vi "Main Data Log.vi"(8 "error in (no error)":errorcluster, 11 "main ref":T1) -> (0 "error out":errorcluster)   [LabVIEW 2025]
uses:
  controls/LAB-IQ UI Data.ctl
panel:
  out "error out 2":errorcluster
  out "TDMS CLOSE":bool
  out "tdms file out":refnum<k34>
  out "File Create Temp":bool
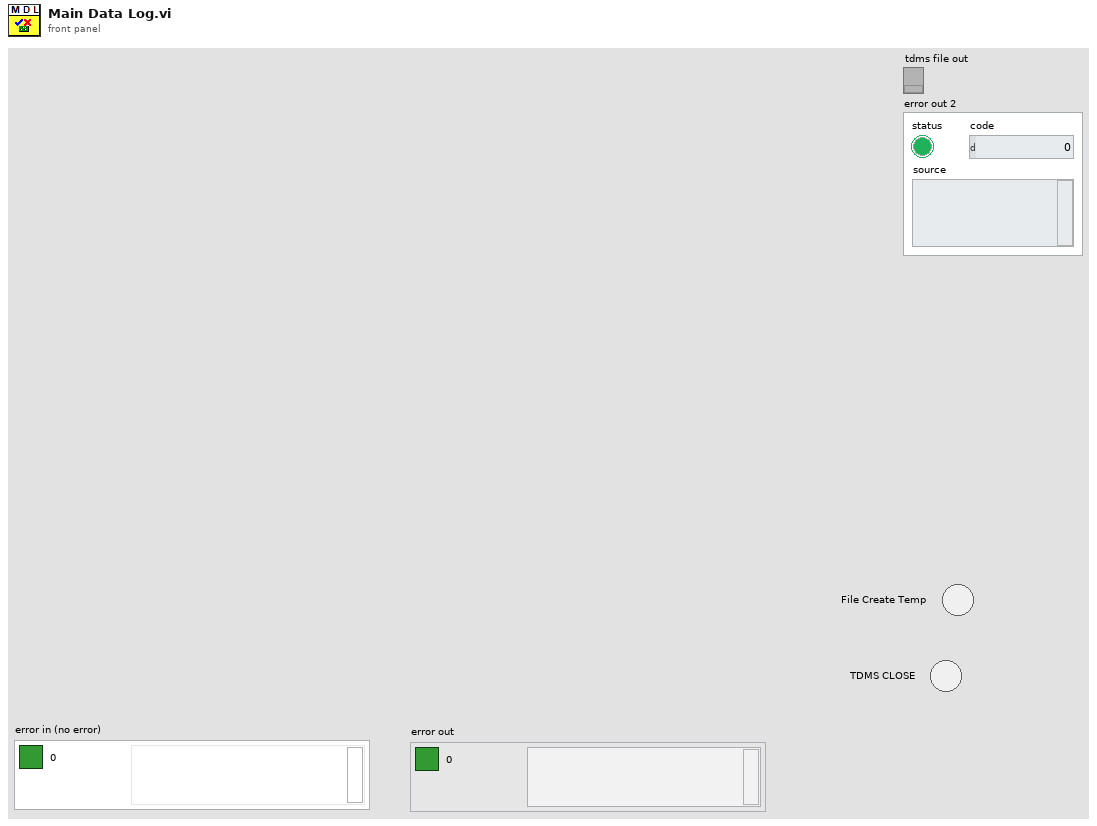
[diagram p1: front panel]
types:
  T1 = typedef "LAB-IQ UI Data.ctl" = cluster{"Main Home Screen":cluster{"GUI":refnum<vi>, "Platform Settings":refnum<vi>, "Configure":refnum<vi>, "Home":refnum<vi>, "EXIT":refnum<vi>, "service 2":refnum<vi>, "MainPage":refnum<vi>, "Analysis":refnum<vi>}, "Platform Settings":cluster{"mm/s  Surge":refnum<vi>, "Update Surge Speed":refnum<vi>, "Drive Error":refnum<vi>, "Disable Axis Jog Soft Limits":refnum<vi>, "mm/s  Sway":refnum<vi>, "Sway and Surge COM Status":refnum<vi>, "Heave COM Status":refnum<vi>, "Enable Platform":refnum<vi>, "Surge Forward Main":refnum<vi>, "Sway Right Main":refnum<vi>, "Sway Left Main":refnum<vi>, "Heave Down Main":refnum<vi>, "Heave Up main":refnum<vi>, "Update Sway Speed":refnum<vi>, "Update Heave Speed":refnum<vi>, "mm/s Heave":refnum<vi>, "mm/sec":refnum<vi>, "mm":refnum<vi>, "Surge Backward Main":refnum<vi>}, "Analysis Screen":cluster{"Analysis Home":refnum<vi>, "Surface Analysis":refnum<vi>, "Imaging":refnum<vi>, "Image Analysis":refnum<vi>, "Post Analysis":refnum<vi>}, "Config Screen":cluster{"Select Load Head":refnum<vi>, "Notes :":refnum<vi>, "FILE":refnum<vi>, "Sample ID :":refnum<vi>, "Operator ID :":refnum<vi>, "Operator Name :":refnum<vi>, "Auto":refnum<vi>}, "Motion Module":cluster{"zNL":refnum<vi>, "NL disp":refnum<vi>, "Rotary Tab":refnum<vi>, "Motion Direction:  3":refnum<vi>, "E.Velocity 2":refnum<vi>, "e.v/ssr 2":refnum<vi>, "Enter Fixed E.Velocity 2":refnum<vi>, "Enter Final SRR 2":refnum<vi>, "Enter initial SRR 2":refnum<vi>, "Enter Fixed SRR 2":refnum<vi>, "Enter the Final E.Velocity (m/s) 2":refnum<vi>, "Enter initial E.Velocity (m/s) 2":refnum<vi>, "Final Speed (RPM) 3":refnum<vi>, "Initial Speed (RPM) 2":refnum<vi>, "Enter the Final Velocity (m/s) 3":refnum<vi>, "Enter initial Velocity (m/s)  3":refnum<vi>, "Ramp Up 2":refnum<vi>, "TEST SELECTION":refnum<vi>, "SPEED SELECTION : ":refnum<vi>, "Angular Oscillation Set":refnum<vi>, "Traction":refnum<vi>, "Step Speed":refnum<vi>, "StepTable For Load-Speed":refnum<vi>, "StepTable For Speed":refnum<vi>, "Surge Forward MM":refnum<vi>, "Surge Backward MM":refnum<vi>, "M3 Image":refnum<vi>, "String 39":refnum<vi>, "Sway Left MM":refnum<vi>, "Sway Right MM":refnum<vi>, "Disable Axis Jog Soft Limits":refnum<vi>, "mm":refnum<vi>, "Heave Down MM":refnum<vi>, "Heave Up MM":refnum<vi>, "Wear Track Diameter (mm)":refnum<vi>, "Set WTD":refnum<vi>, "HomeScratch":refnum<vi>, "HomeRot":refnum<vi>, "PlaceModule":refnum<vi>, "Enter the Angle (Deg)":refnum<vi>, "Enter the Frequency (Hz)":refnum<vi>, "Motion Mode:":refnum<vi>, "LR Sway":refnum<vi>, "Rot Hor":refnum<vi>, "Scratch":refnum<vi>, "LR Cam":refnum<vi>, "MMBack":refnum<vi>, "MMNext":refnum<vi>, "Rot Ver":refnum<vi>, "Rotary Module Selection":refnum<vi>, "calculate rotary":refnum<vi>, "SPEED SELECTION : rotary":refnum<vi>, "Import 2":refnum<vi>, "Save 2":refnum<vi>, "File Path :  2":refnum<vi>, "String 45":refnum<vi>, "StepTable For Speed 3":refnum<vi>, "Enter the Speed(mm/sec)":refnum<vi>, "Enter the Speed(RPM)":refnum<vi>, "Enter Scratch Speed (mm/s):":refnum<vi>, "SwaySpeed Set":refnum<vi>, "Scartch Offset":refnum<vi>, "Motion type:":refnum<vi>, "HomeScratch 2":refnum<vi>, "Enter Scratch length (mm):":refnum<vi>, "Wear Track Diameter":refnum<vi>, "Rotary Speed Exced":refnum<vi>, "Scratch Mode":refnum<vi>, "No of Scratch":refnum<vi>}, "Environmental control":cluster{"Humidity  Status  3":refnum<vi>, "Low Temp  Status  2":refnum<vi>, "TK4 status 2":refnum<vi>, "Stage Temperature":refnum<vi>, "Sample Temperature":refnum<vi>, "Humidity (Amb)":refnum<vi>, "Clear List":refnum<vi>, "Add to list":refnum<vi>, "Wear":refnum<vi>, "Vibration":refnum<vi>, "Humidity (Chamber)":refnum<vi>, "Temperature (Chamber)":refnum<vi>, "ECR ":refnum<vi>, "Temperature (Amb)":refnum<vi>, "Microphone":refnum<vi>, "Acoustic Emission 3":refnum<vi>, "SNext":refnum<vi>, "APBack":refnum<vi>, "Enter the Temperature (°C):":refnum<vi>, "Enter the Stage \nTemperature (°C):":refnum<vi>, "Enter the Humidity (%Rh):":refnum<vi>, "Low Temp":refnum<vi>, "High Temp":refnum<vi>, "Humidity":refnum<vi>, "Sensors Picked":refnum<vi>}, "About Screen":cluster{"Password":refnum<vi>, "Home Service":refnum<vi>, "Advanced Setting":refnum<vi>, "About Tab":refnum<vi>, "ECR Port:":refnum<vi>, "Ramp Port:":refnum<vi>, "Installation/Replacement completed":refnum<vi>, "Loahead":refnum<vi>, "Heave and Surge COM Port:":refnum<vi>, "Sway COM Port:":refnum<vi>, "Temp Modbus:":refnum<vi>, "Humidity Port:":refnum<vi>, "Edit Gain Constants":refnum<vi>, "Save Gain Constants":refnum<vi>}, "Main Screen":cluster{"Main Screen Tab":refnum<vi>, "Angle and Frequency":refnum<vi>, "Stroke (mm)":refnum<vi>, "Angle (Deg)":refnum<vi>, "Main Speed Tab":refnum<vi>, "MTM MOTOR DISPLAY":refnum<vi>, "Disc Speed (m/sec)":refnum<vi>, "Ball Speed (m/sec)":refnum<vi>, "Disc Speed (RPM)":refnum<vi>, "Ball Speed (RPM)":refnum<vi>, "SPEED TAB":refnum<vi>, "Speed (m/sec)":refnum<vi>, "Set Speed (m/sec)":refnum<vi>, "Speed (RPM)":refnum<vi>, "Set Speed":refnum<vi>, "Time Tab":refnum<vi>, "Time ( HH:MM:SS ) 2":refnum<vi>, "Test Duration":refnum<vi>, "Test Duration 4":refnum<vi>, "TEST CYCLE":refnum<vi>, "TOTAL CYCLES":refnum<vi>, "Set Load (N)":refnum<vi>, "Temp Tabs":refnum<vi>, "Heater":refnum<vi>, "TK4 status":refnum<vi>, "ChamberTemp":refnum<vi>, "SetTmp":refnum<vi>, "Controller  Status":refnum<vi>, "ChamberTemp 2":refnum<vi>, "SetTmp 2":refnum<vi>, "Controller  Status 2":refnum<vi>, "ChamberTemp 3":refnum<vi>, "SetTmp 3":refnum<vi>, "Cooling":refnum<vi>, "Load Communication":refnum<vi>, "Ambient \nTemperature":refnum<vi>, "HumCOMStatus":refnum<vi>, "Ambient\n Humidity":refnum<vi>, "Freq (Hz)":refnum<vi>, "Load En":refnum<vi>, "NLt":refnum<vi>, "zNL 2":refnum<vi>, "Humidity On":refnum<vi>, "humidity disp":refnum<vi>, "Set Humidity":refnum<vi>, "NL disp 2":refnum<vi>, "Humidity On 2":refnum<vi>, "humidity disp 2":refnum<vi>, "Set Humidity 2":refnum<vi>, "NL disp 3":refnum<vi>, "AppLoadSeq scratch":refnum<vi>, "Stop Scratch":refnum<vi>, "ClrLog":refnum<vi>, "Trip Log":refnum<vi>, "STOP":refnum<vi>, "Start Test":refnum<vi>, "Test status":refnum<vi>, "AR Led":refnum<vi>, "Data":refnum<vi>, "Health":refnum<vi>, "Sway COM Status":refnum<vi>, "Heave COM Status":refnum<vi>, "Grp Tab":refnum<vi>, "Sub Graph":refnum<vi>, "SD (mm)":refnum<vi>, "Siliding distance Reset Graph":refnum<vi>, "SDGp":refnum<vi>, "Humidity Reset Graph":refnum<vi>, "HumrGp":refnum<vi>, "Acoustic Emission (mV)":refnum<vi>, "Aqucostic Reset Graph":refnum<vi>, "gACQUOS":refnum<vi>, "ECR RESET":refnum<vi>, "ECR":refnum<vi>, "Temperature Reset":refnum<vi>, "Acoustic Emission (mV) 2":refnum<vi>, "Aqucostic Reset Graph 2":refnum<vi>, "gACQUOS 2":refnum<vi>, "ECR RESET 2":refnum<vi>, "ECR 2":refnum<vi>, "Temperature Reset 2":refnum<vi>, "Temperature (deg c)":refnum<vi>, "Speed Reset Graph":refnum<vi>, "Speed Tab":refnum<vi>, "MTM DISC  SPEED":refnum<vi>, "MTM BALL SPEED":refnum<vi>, "speed mm/sec":refnum<vi>, "Hymidity":refnum<vi>, "Humidity Disable trip":refnum<vi>, "CoF Trip  2":refnum<vi>, "Depth Trip":refnum<vi>, "Weart Deapth":refnum<vi>, "Depth Reset Graph":refnum<vi>, "Weart":refnum<vi>, "Depthz":refnum<vi>, "Depth (µm)":refnum<vi>, "WearGp":refnum<vi>, "NL Trip 2":refnum<vi>, "Load pid":refnum<vi>, "Load Disable Trip":refnum<vi>, "Load Reset Graph":refnum<vi>, "NL Display 4":refnum<vi>, "Main Chart 3":refnum<vi>, "BACK":refnum<vi>, "Depth Trip 2":refnum<vi>, "COF TRIP ":refnum<vi>, "Friction Force (N)":refnum<vi>, "FF Reset Graph":refnum<vi>, "FF Disable Trip":refnum<vi>, "FF TRIP":refnum<vi>, "COF Disable Trip":refnum<vi>, "COF Reset Graph":refnum<vi>, "Start Test Temp":refnum<vi>, "zFF":refnum<vi>, "Friction Force (N) Graph":refnum<vi>, "Coefficient of Friction":refnum<vi>, "Scratch Start Test":refnum<vi>, "FF Tab":refnum<vi>, "Cyclic Friction Force (N)":refnum<vi>, "CZ FF":refnum<vi>, "Cyclic Friction Force (N) Graph":refnum<vi>, "Cyclic Coefficient of Friction":refnum<vi>, "Cyclic FF TRIP":refnum<vi>, "Cyclic FF Disable Trip":refnum<vi>, "cyclic COF Disable Trip":refnum<vi>, "cyclic COF TRIP":refnum<vi>, "cyclic COF Reset Graph":refnum<vi>, "Cyclic FF Reset Graph":refnum<vi>, "Test Trip":refnum<vi>, "Multi Scratch Pass":refnum<vi>, "Scratch Start Recording":refnum<vi>}, "Loading":cluster{"Indentation":refnum<vi>, "Reference Sample":refnum<vi>, "Load Cell Communication Slide":refnum<vi>, "com 3":refnum<vi>, "com":refnum<vi>, "DecaForce COM Status":refnum<vi>, "Update":refnum<vi>, "Clear 3":refnum<vi>, "seq":refnum<vi>, "Stribeck table":refnum<vi>, "Stribeck Table  For loading":refnum<vi>, "Loading Mode":refnum<vi>, "Enter the Final Load (N)":refnum<vi>, "Enter the CoF Trip":refnum<vi>, "Enter the Friction Force Trip":refnum<vi>, "Enter the Normal load Trip":refnum<vi>, "Enter the Load  (N)":refnum<vi>, "KiloForce":refnum<vi>, "DecaForce ":refnum<vi>, "MicroForce":refnum<vi>, "LHBack":refnum<vi>, "LHNext":refnum<vi>, "Enter the Loading Rate (N/min)":refnum<vi>, "Message":refnum<vi>, "Warning 2":refnum<vi>, "SSP 0.75":refnum<vi>, "SSP 0.5":refnum<vi>, "SSP 0.3":refnum<vi>, "Warning":refnum<vi>, "gui GIF":refnum<vi>, "Communication is established":refnum<vi>, "AppLoad 4":refnum<vi>, "Multipoint":refnum<vi>, "Load Selection":refnum<vi>}, "PID":cluster{"Ramp MulFac":refnum<vi>, "pulses LoadDiffRamp(2..10)":refnum<vi>, "PulseControlRamp(diff<=3N)":refnum<vi>, "SetLoadDeadband(%) Load(0-10N)":refnum<vi>, "PID gains out delay (microForce)":refnum<vi>, "Ramp":refnum<vi>, "Gain 2":refnum<vi>, "pulses LoadDiff(2..10)":refnum<vi>, "pulses LoadDiff(11..50)":refnum<vi>, "PulseControl(diff<=3N)":refnum<vi>, "SetLoadDeadband(%)  2":refnum<vi>, "Dummy Run":refnum<vi>, "Vertical load (N)":refnum<vi>, "AutoTune":refnum<vi>, "Offset 3 ":refnum<vi>, "apply load":refnum<vi>, "Offset  3":refnum<vi>, "apply load 2":refnum<vi>, "Enter ByPass Load":refnum<vi>, "reinit 3":refnum<vi>, "output range delay":refnum<vi>, "PID gains out delay":refnum<vi>, "Bypass Load":refnum<vi>, "pulsesSent":refnum<vi>, "pulses ":refnum<vi>, "actpid":refnum<vi>, "gFF Rot":refnum<vi>, "pulses LoadDiff(21..1000)":refnum<vi>, "Delay":refnum<vi>, "deadband":refnum<vi>}, "Config Parameters":cluster{"Tab Control 3":refnum<vi>, "Tab Control 19":refnum<vi>, "SAMPLES":refnum<vi>, "Re-initilaize":refnum<vi>, "Filter ON/OFF":refnum<vi>, "TracHomeSurgeOffsetCounts 10MM":refnum<vi>, "TracHomeSwayOffsetCounts 10MM":refnum<vi>, "Acoustic Emission:":refnum<vi>, "Apply Filter (FF)":refnum<vi>, "Filter% 2":refnum<vi>, "Apply Filter (Load)":refnum<vi>, "Filter% ":refnum<vi>, "Sway distance (mm)":refnum<vi>, "Surge distance (mm)":refnum<vi>, "DataSavingLoopDelay(ms)":refnum<vi>, "SAVE 2":refnum<vi>, "Enter Distance":refnum<vi>, "Sway Counts:":refnum<vi>, "Distance (mm): 3":refnum<vi>, "Surge Counts:":refnum<vi>, "Distance (mm): 2":refnum<vi>, "Distance (mm):":refnum<vi>, "Heave Counts:":refnum<vi>, "LRMHomeSurgeOffsetCounts":refnum<vi>, "LRMHomeSwayOffsetCounts":refnum<vi>, "TracHomeSurgeOffsetCounts 20MM":refnum<vi>, "TracHomeSwayOffsetCounts 20MM":refnum<vi>, "RotHomeSwayOffsetCounts":refnum<vi>, "RotHomeSurgeOffsetCounts":refnum<vi>, "Heave distance":refnum<vi>, "Zmm":refnum<vi>, "Heave Pulses/mm":refnum<vi>, "Surge Pulses/mm":refnum<vi>, "Sway Pulses/mm":refnum<vi>, "Heave Pitch":refnum<vi>, "Surge Pitch":refnum<vi>, "Sway Pitch":refnum<vi>, "Heave PPR":refnum<vi>, "Surge PPR":refnum<vi>, "Sway PPR":refnum<vi>, "Tab Control 5":refnum<vi>, "Tab Control 14":refnum<vi>, "Tab Control 26":refnum<vi>, "AE":refnum<vi>, "Heave Loop Delay":refnum<vi>, "Heave PID Speed":refnum<vi>, "Surge Jog Speed":refnum<vi>, "Heave Jog Speed":refnum<vi>, "Sway Loop Delay":refnum<vi>, "Sway PID Speed":refnum<vi>, "Sway Jog Speed":refnum<vi>, "DEPTH TRIP VALUE":refnum<vi>, "LOAD TRIP VALUE":refnum<vi>, "DEPTH TRIP   ENABLE":refnum<vi>, "LOAD TRIP  ENABLE":refnum<vi>, "CYCLIC FF TRIP VALUE":refnum<vi>, "FF TRIP VALUE":refnum<vi>, "CYCLIC CoF TRIP VALUE":refnum<vi>, "COF TRIP VALUE":refnum<vi>, "CYCLIC COF TRIP  ENABLE":refnum<vi>, "CYCLIC FF TRIP  ENABLE":refnum<vi>, "FF TRIP  ENABLE":refnum<vi>, "COF TRIP  ENABLE":refnum<vi>}, "Loading Com Port":cluster{"ClearAll":refnum<vi>, "Mz(Nm)":refnum<vi>, "My(Nm)":refnum<vi>, "Mx(Nm)":refnum<vi>, "Save Dwell":refnum<vi>, "Mx ":refnum<vi>, "My ":refnum<vi>, "Mz":refnum<vi>, "Fx(N)":refnum<vi>, "Fy(N)":refnum<vi>, "Fz(N)":refnum<vi>, "ZeroAll":refnum<vi>, "Acq Delay (ms)":refnum<vi>, "Burst Delay (ms)":refnum<vi>, "model":refnum<vi>, "SN":refnum<vi>, "FFx(N)":refnum<vi>, "Sensor IP":refnum<vi>, "Port":refnum<vi>, "FFy(N)":refnum<vi>, "Load(N)":refnum<vi>, "delete Handle":refnum<vi>, "Create Handle":refnum<vi>, "ft_data":refnum<vi>, "ft_range":refnum<vi>, "ft_data 2":refnum<vi>, "stop 6":refnum<vi>, "running_flag":refnum<vi>, "ft_udp_handle":refnum<vi>, "get-data-return":refnum<vi>, "get-range-return":refnum<vi>, "zero-return":refnum<vi>, "filter-return":refnum<vi>, "initial-return":refnum<vi>, "deleteHandle-result":refnum<vi>, "Load Cell Temp":refnum<vi>}, "Heave AND Surge":cluster{"SURGE POSE":refnum<vi>, "error out Read":refnum<vi>, "HEAVE POSE":refnum<vi>, "State":refnum<vi>, "Homed":refnum<vi>, "Sequence ID":refnum<vi>, "error out Write":refnum<vi>, "faultCode":refnum<vi>, "Ack ID":refnum<vi>, "SPEED":refnum<vi>, "Distance":refnum<vi>, "Mode Command":refnum<vi>, "Heave and Surge Read":refnum<vi>, "Read Heave Temp":refnum<vi>, "Spare 15":refnum<vi>, "Spare 14":refnum<vi>, "Spare 13":refnum<vi>, "Spare 12":refnum<vi>, "Spare 11":refnum<vi>, "Spare 10":refnum<vi>, "Spare 9":refnum<vi>, "Spare 8":refnum<vi>, "Spare 7":refnum<vi>, "Spare 6":refnum<vi>, "Spare 5":refnum<vi>, "Spare 4":refnum<vi>, "Spare 2":refnum<vi>, "Spare 1":refnum<vi>, "Node Id":refnum<vi>, "Spare 3":refnum<vi>, "SPARE 4":refnum<vi>, "SPARE 3":refnum<vi>, "SPARE 2":refnum<vi>, "SPARE 1":refnum<vi>, "fwMajor":refnum<vi>, "fwMinor":refnum<vi>, "Manual Write":refnum<vi>, "Heave and Surge Write":refnum<vi>}, "New PID LOGIC":cluster{"Fine Tune Zone":refnum<vi>, "PID SDelay":refnum<vi>, "Max_pos_limit":refnum<vi>, "Min_pos_limit":refnum<vi>, "i_limit":refnum<vi>, "pct_scale":refnum<vi>, "Deadband":refnum<vi>, "Kd":refnum<vi>, "Ki":refnum<vi>, "Kp":refnum<vi>, "Current Position":refnum<vi>, "Set Load":refnum<vi>, "Current Load":refnum<vi>, "Pulse delta":refnum<vi>, "Init Step":refnum<vi>, "Max Step Linit":refnum<vi>}, "SWAY ":cluster{"fwMajor":refnum<vi>, "Homed":refnum<vi>, "Rotary POSE":refnum<vi>, "State":refnum<vi>, "SWAY POSE":refnum<vi>, "Ack ID":refnum<vi>, "faultCode":refnum<vi>, "Node Id":refnum<vi>, "fwMinor":refnum<vi>, "Spare 6":refnum<vi>, "Spare 5":refnum<vi>, "Spare 4":refnum<vi>, "Spare 3":refnum<vi>, "Spare 2":refnum<vi>, "Spare 1":refnum<vi>, "Spare 7":refnum<vi>, "SPARE  5":refnum<vi>, "error out Write  SWAY ":refnum<vi>, "error out Read SWAY ":refnum<vi>, "Manual Write SWAY ":refnum<vi>, "SWAY WRITE":refnum<vi>, "SPARE  4":refnum<vi>, "SPARE  3":refnum<vi>, "SPARE 2":refnum<vi>, "SPARE 1":refnum<vi>, "Spare 15":refnum<vi>, "Spare 14":refnum<vi>, "Spare 13":refnum<vi>, "Spare 12":refnum<vi>, "Spare 11":refnum<vi>, "Spare 9":refnum<vi>, "Spare 8":refnum<vi>, "SPEED":refnum<vi>, "Distance":refnum<vi>, "Mode Command":refnum<vi>, "Sequence ID":refnum<vi>, "SWAY READ":refnum<vi>, "Spare 10":refnum<vi>, "Read SWAY Temp":refnum<vi>}, "Analysis Screen":cluster{"Analysis Home":refnum<vi>, "Refresh 2":refnum<vi>, "MEAN 4":refnum<vi>, "SD 4":refnum<vi>, "VARIANCE 4":refnum<vi>, "MEAN  3":refnum<vi>, "SD  3":refnum<vi>, "VARIANCE  3":refnum<vi>, "MEAN 2":refnum<vi>, "SD  2":refnum<vi>, "VARIANCE 2":refnum<vi>, "MEAN":refnum<vi>, "SD":refnum<vi>, "VARIANCE":refnum<vi>, "File 4 Discription":refnum<vi>, "OPEN 4":refnum<vi>, "File Name 4":refnum<vi>, "OPEN 3":refnum<vi>, "File 3 Discription":refnum<vi>, "File Name 3":refnum<vi>, "Y-AXIS":refnum<vi>, "X-AXIS":refnum<vi>, "XY Graph":refnum<vi>, "File Name 2":refnum<vi>, "File Name 1":refnum<vi>, "OPEN 2":refnum<vi>, "OPEN 1":refnum<vi>, "File 1 Discription ":refnum<vi>, "File 2 Discription":refnum<vi>, "Export":refnum<vi>, "File Format":refnum<vi>}}
  T2 = enum32{"  Acquire  ", "Compare Files Rot", "About", "Service"}
  T3 = enum32{"Setup", "Load Head", "Motion Module", "Environment", "Begin"}
  T4 = enum16{"open", "open or create", "create or replace", "create", "open (read-only)"}
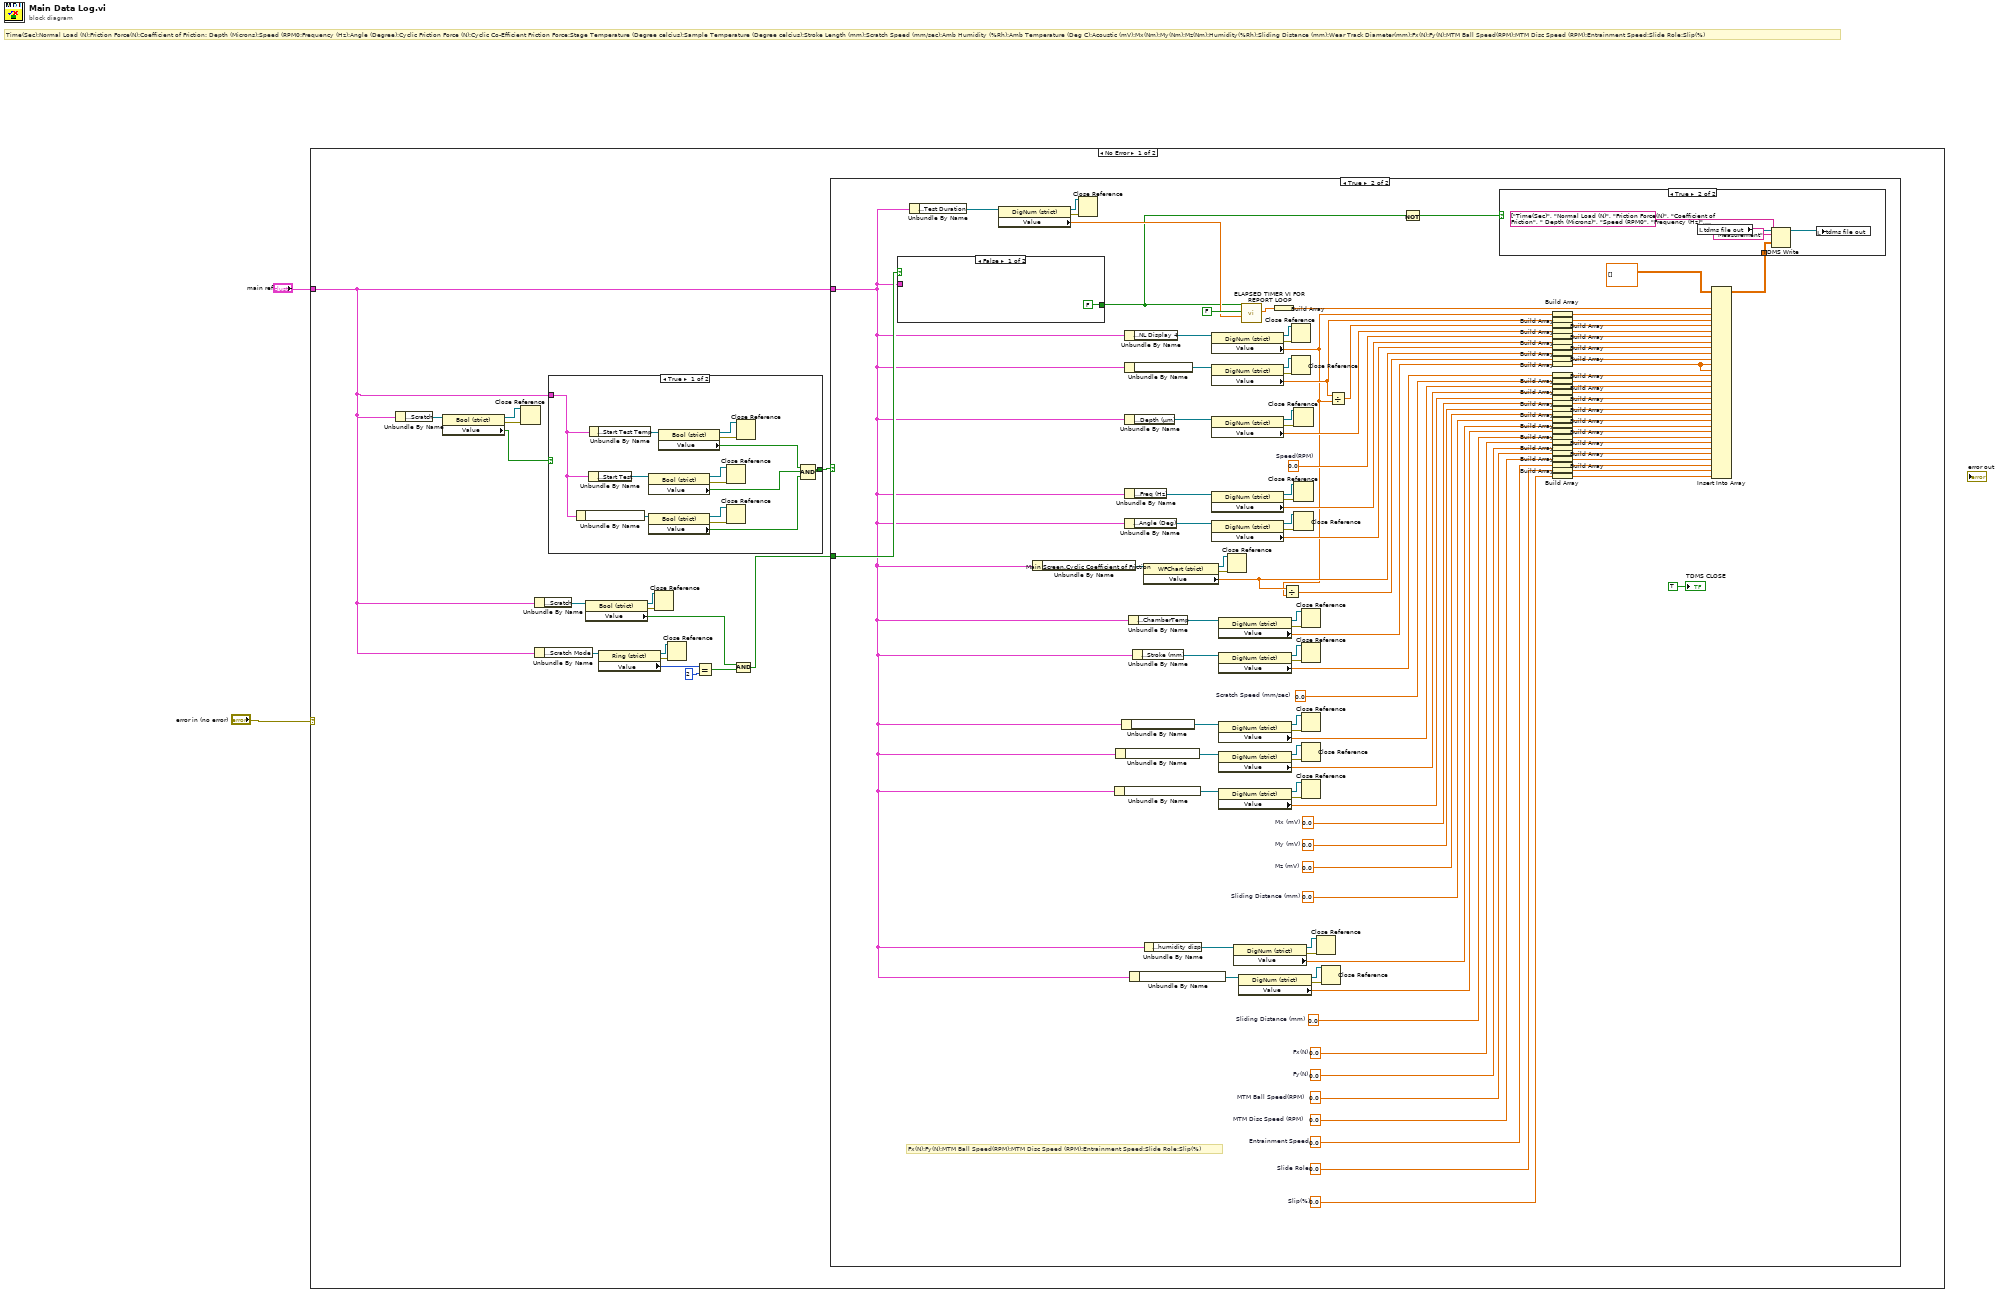
[diagram p0: block diagram]
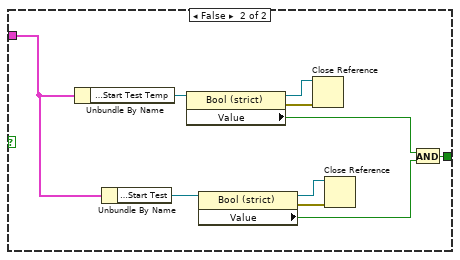
[diagram p2: hidden frame]
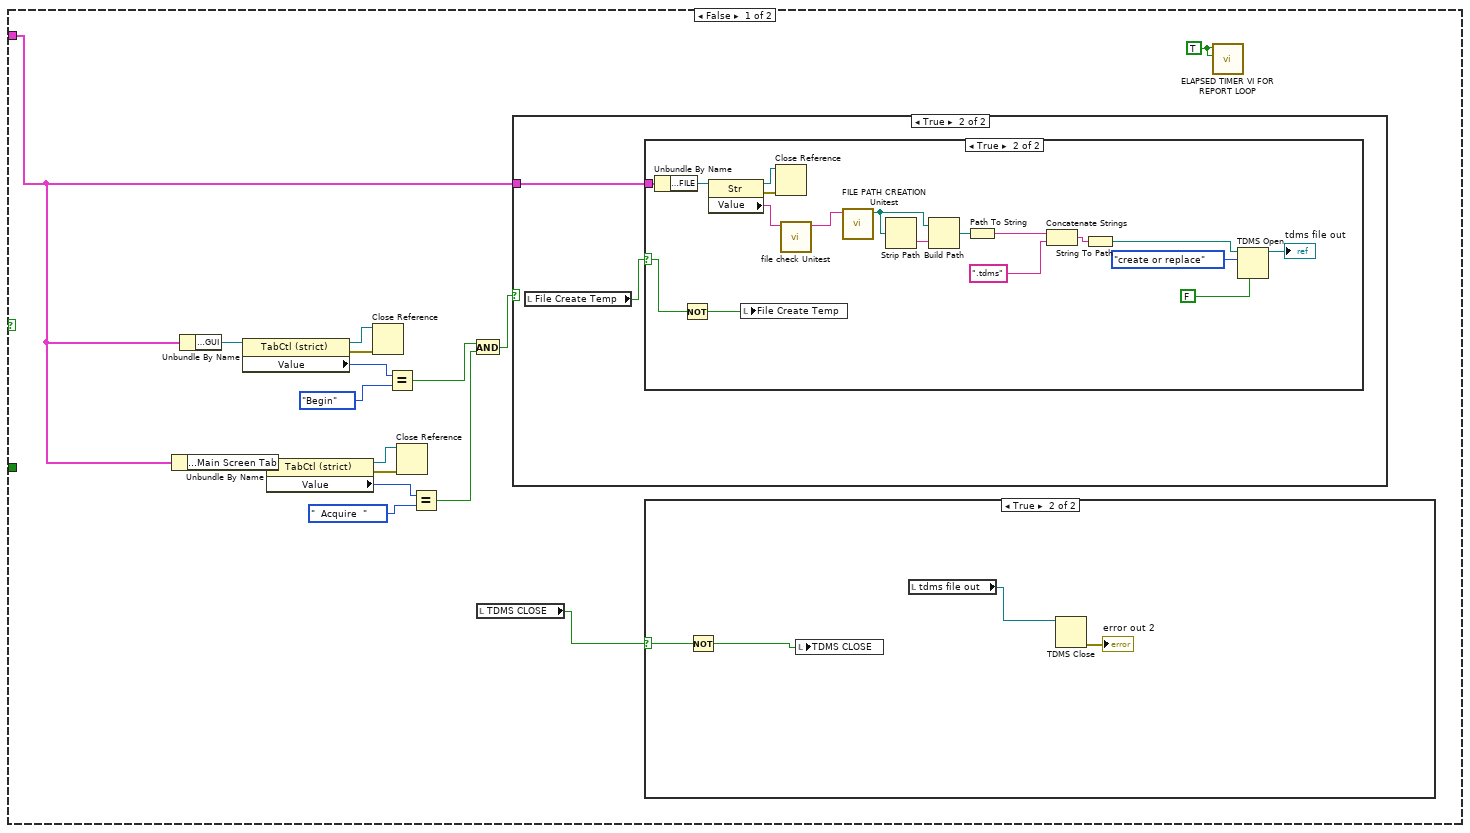
[diagram p3: hidden frame]
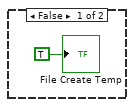
[diagram p5: hidden frame]
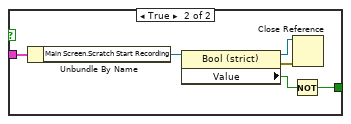
[diagram p7: hidden frame]
diagram:
  # "Time(Sec):Normal Load (N):Friction Force(N):Coefficient of Friction: Depth (Microns):Speed (RPM0:Frequency (Hz):Angle (Degree):Cyclic Friction Force (N):Cyclic Co-Efficient Friction Force:Stage Temperature (Degree celcius):Sample Temperature (Degree celcius):Stroke Length (mm):Scratch Speed (mm/sec):Amb Humidity (%Rh):Amb Temperature (Deg C):Acoustic (mV):Mx(Nm):My(Nm);Mz(Nm):Humidity(%Rh):Sliding Distance (mm):Wear Track Diameter(mm):Fx(N):Fy(N):MTM Ball Speed(RPM):MTM Disc Speed (RPM):Entrainment Speed:Slide Role:Slip(%)"
  n1 = case shown="No Error" "error in (no error)" {
    tunnel: "main ref" -> [w4 _]
    frame No Error {
      n2 = Unbundle By Name(w4) -> ("Motion Module.Scratch"=w18:refnum<vi>)
      n3 = property class="Bool (strict)"(reference=w18) -> (reference out=w19:refnum<vi>, error out=w17:errorcluster, "Value"=w16:bool)  [unwired: 1 in]
      n4 = Close Reference(reference=w19, error in (no error)=w17) -> ()  [unwired: 1 out]
      n5 = Unbundle By Name(w4) -> ("Motion Module.Scratch"=w13:refnum<vi>)
      n6 = Unbundle By Name(w4) -> ("Motion Module.Scratch Mode"=w10:refnum<vi>)
      n7 = case shown="True" w16 {
        tunnel: w4 -> [w21 w37]
        tunnel: [w25 w34] -> w15
        frame True {
          n8 = Unbundle By Name(w21) -> ("Main Screen.Scratch Start Test"=w23:refnum<vi>)
          n9 = Unbundle By Name(w21) -> ("Main Screen.Start Test"=w29:refnum<vi>)
          n10 = Unbundle By Name(w21) -> ("Main Screen.Start Test Temp"=w32:refnum<vi>)
          n11 = property class="Bool (strict)"(reference=w29) -> (reference out=w28:refnum<vi>, error out=w30:errorcluster, "Value"=w26:bool)  [unwired: 1 in]
          n12 = property class="Bool (strict)"(reference=w23) -> (reference out=w24:refnum<vi>, error out=w22:errorcluster, "Value"=w20:bool)  [unwired: 1 in]
          n13 = property class="Bool (strict)"(reference=w32) -> (reference out=w33:refnum<vi>, error out=w31:errorcluster, "Value"=w27:bool)  [unwired: 1 in]
          n14 = Close Reference(reference=w28, error in (no error)=w30) -> ()  [unwired: 1 out]
          n15 = Close Reference(reference=w24, error in (no error)=w22) -> ()  [unwired: 1 out]
          n16 = Close Reference(reference=w33, error in (no error)=w31) -> ()  [unwired: 1 out]
          n17 = Compound Arithmetic op=AND(w27, w26, w20) -> (w25:bool)
        }
        frame False {
          n18 = Unbundle By Name(w37) -> ("Main Screen.Start Test Temp"=w42:refnum<vi>)
          n19 = Unbundle By Name(w37) -> ("Main Screen.Start Test"=w39:refnum<vi>)
          n20 = property class="Bool (strict)"(reference=w42) -> (reference out=w43:refnum<vi>, error out=w41:errorcluster, "Value"=w36:bool)  [unwired: 1 in]
          n21 = property class="Bool (strict)"(reference=w39) -> (reference out=w38:refnum<vi>, error out=w40:errorcluster, "Value"=w35:bool)  [unwired: 1 in]
          n22 = Close Reference(reference=w43, error in (no error)=w41) -> ()  [unwired: 1 out]
          n23 = Close Reference(reference=w38, error in (no error)=w40) -> ()  [unwired: 1 out]
          n24 = And(x=w36, y=w35) -> (x .and. y?=w34:bool)
        }
      }
      n25 = property class="Bool (strict)"(reference=w13) -> (reference out=w12:refnum<vi>, error out=w14:errorcluster, "Value"=w5:bool)  [unwired: 1 in]
      n26 = property class="Ring (strict)"(reference=w10) -> (reference out=w11:refnum<vi>, error out=w9:errorcluster, "Value"=w8:u16)  [unwired: 1 in]
      n27 = Close Reference(reference=w12, error in (no error)=w14) -> ()  [unwired: 1 out]
      n28 = Close Reference(reference=w11, error in (no error)=w9) -> ()  [unwired: 1 out]
      n29 = Equal?(x=w8, y=u16 2) -> (x = y?=w6:bool)
      n30 = Compound Arithmetic op=AND(w5, w6) -> (w3:bool)
      n31 = case shown="True" w15 {
        tunnel: w4 -> [w49 w87]
        tunnel: w3 -> [_ w88]
        frame False {
          w59 = TRUE ("PAUSE")
          n32 = Unbundle By Name(w49) -> ("Main Screen.Main Screen Tab"=w51:refnum<vi>)
          n33 = Unbundle By Name(w49) -> ("Main Home Screen.GUI"=w57:refnum<vi>)
          n34 = property class="TabCtl (strict)"(reference=w57) -> (reference out=w56:refnum<vi>, error out=w58:errorcluster, "Value"=w55:T3)  [unwired: 1 in]
          n35 = property class="TabCtl (strict)"(reference=w51) -> (reference out=w52:refnum<vi>, error out=w50:errorcluster, "Value"=w53:T2)  [unwired: 1 in]
          n36 = Close Reference(reference=w56, error in (no error)=w58) -> ()  [unwired: 1 out]
          n37 = Equal?(x=w55, y=T3."Begin" ("Value")) -> (x = y?=w47:bool)
          n38 = Close Reference(reference=w52, error in (no error)=w50) -> ()  [unwired: 1 out]
          n39 = Equal?(x=w53, y=T2."  Acquire  " ("Value")) -> (x = y?=w46:bool)
          n40 = And(x=w47, y=w46) -> (x .and. y?=w45:bool)
          n41 = local read "TDMS CLOSE"() -> (w44:bool)
          n42 = case shown="True" w45 {
            tunnel: w49 -> [_ w66]
            frame False {
              "File Create Temp" <- TRUE ("File Create Temp")
            }
            frame True {
              n43 = local read "File Create Temp"() -> (w65:bool)
              n44 = case shown="True" w65 {
                selector: w65 -> [_ w74]
                tunnel: w66 -> [_ w75]
                frame False {
                }
                frame True {
                  n45 = Unbundle By Name(w75) -> ("Config Screen.FILE"=w76:refnum<vi>)
                  n46 = Not(x=w74) -> (.not. x?=w73:bool)
                  n47 = property class="Str"(reference=w76) -> (reference out=w78:refnum<vi>, error out=w77:errorcluster, "Value"=w68:string)  [unwired: 1 in]
                  n48 = local write "File Create Temp"(w73) -> ()
                  n49 = Close Reference(reference=w78, error in (no error)=w77) -> ()  [unwired: 1 out]
                  n50 = call "file check Unitest.vi"("file name in"=w68) -> ("file name out"=w67:string)  [unwired: 9 in, 1 out]
                  n51 = call "FILE PATH CREATION Unitest.vi"("FILE NAME :"=w67) -> ("FILE OUT"=w79:path)  [unwired: 9 in, 1 out]
                  n52 = Strip Path(path=w79) -> (name=w82:string)  [unwired: 1 out]
                  n53 = Build Path(base path=w79, name or relative path=w82) -> (appended path=w83:path)
                  n54 = Path To String(path=w83) -> (string=w80:string)
                  n55 = Concatenate Strings(w80, ".tdms" ("string")) -> (w81:string)
                  n56 = String To Path(string=w81) -> (path=w70:path)
                  n57 = TDMS Open(6:FALSE ("disable buffering (T)"), 10:T4."create or replace" ("operation"), 11:w70) -> (3:→"tdms file out":refnum<k34>)  [unwired: 4 in, 1 out]
                }
              }
            }
          }
          n58 = case shown="True" w44 {
            selector: w44 -> [_ w63]
            frame False {
            }
            frame True {
              n59 = Not(x=w63) -> (.not. x?=w62:bool)
              n60 = local write "TDMS CLOSE"(w62) -> ()
              n61 = local read "tdms file out"() -> (w61:refnum<k34>)
              n62 = TDMS Close(11:w61) -> (0:→"error out 2":errorcluster)  [unwired: 1 in, 1 out]
            }
          }
          n63 = call "ELAPSED TIMER VI FOR REPORT LOOP.vi"("RESET"=w59, "PAUSE"=w59) -> ()  [unwired: 7 in, 3 out]
        }
        frame True {
          w131 = 0.0  # Slip(%)
          w132 = 0.0  # Slide Role:
          w133 = 0.0  # Entrainment Speed
          w134 = 0.0  # MTM Disc Speed (RPM)
          w135 = 0.0  # MTM Ball Speed(RPM)
          w136 = 0.0  # Fy(N)
          w137 = 0.0  # Fx(N)
          w142 = 0.0  # Mz (mV)
          w143 = 0.0  # My (mV)
          w144 = 0.0  # Mx (mV)
          w138 = 0.0  # Sliding Distance (mm)
          w141 = 0.0  # Sliding Distance (mm)
          w149 = 0.0  # Scratch Speed (mm/sec)
          w172 = 0.0  # Speed(RPM)
          # "Fx(N):Fy(N):MTM Ball Speed(RPM):MTM Disc Speed (RPM):Entrainment Speed:Slide Role:Slip(%)"
          n64 = case shown="False" w88 {
            tunnel: w87 -> [_ w199]
            tunnel: [FALSE ("Value") w197] -> w86
            frame False {
            }
            frame True {
              n65 = Unbundle By Name(w199) -> ("Main Screen.Scratch Start Recording"=w201:refnum<vi>)
              n66 = property class="Bool (strict)"(reference=w201) -> (reference out=w200:refnum<vi>, error out=w202:errorcluster, "Value"=w198:bool)  [unwired: 1 in]
              n67 = Not(x=w198) -> (.not. x?=w197:bool)
              n68 = Close Reference(reference=w200, error in (no error)=w202) -> ()  [unwired: 1 out]
            }
          }
          n69 = Unbundle By Name(w87) -> ("Main Screen.Test Duration"=w128:refnum<vi>)
          n70 = property class="DigNum (strict)"(reference=w128) -> (reference out=w129:refnum<vi>, error out=w130:errorcluster, "Value"=w127:dbl)  [unwired: 1 in]
          n71 = Unbundle By Name(w87) -> ("Main Screen.Cyclic Coefficient of Friction"=w126:refnum<vi>)
          n72 = Close Reference(reference=w129, error in (no error)=w130) -> ()  [unwired: 1 out]
          n73 = Unbundle By Name(w87) -> ("Main Screen.Acoustic Emission (mV)"=w153:refnum<vi>)
          n74 = Unbundle By Name(w87) -> ("Main Screen.Ambient \nTemperature"=w159:refnum<vi>)
          n75 = Unbundle By Name(w87) -> ("Main Screen.Ambient\n Humidity"=w162:refnum<vi>)
          n76 = Unbundle By Name(w87) -> ("Main Screen.NL Display 4"=w192:refnum<vi>)
          n77 = Unbundle By Name(w87) -> ("Main Screen.Friction Force (N)"=w187:refnum<vi>)
          n78 = Unbundle By Name(w87) -> ("Main Screen.Depth (µm)"=w184:refnum<vi>)
          n79 = Unbundle By Name(w87) -> ("Main Screen.Freq (Hz)"=w178:refnum<vi>)
          n80 = Unbundle By Name(w87) -> ("Main Screen.Angle (Deg)"=w177:refnum<vi>)
          n81 = Unbundle By Name(w87) -> ("Main Screen.ChamberTemp"=w173:refnum<vi>)
          n82 = Unbundle By Name(w87) -> ("Motion Module.Wear Track Diameter (mm)"=w156:refnum<vi>)
          n83 = Unbundle By Name(w87) -> ("Main Screen.Stroke (mm)"=w166:refnum<vi>)
          n84 = property class="WFChart (strict)"(reference=w126) -> (reference out=w121:refnum<vi>, error out=w125:errorcluster, "Value"=w124:dbl)  [unwired: 1 in]
          n85 = Unbundle By Name(w87) -> ("Main Screen.humidity disp"=w152:refnum<vi>)
          n86 = property class="DigNum (strict)"(reference=w192) -> (reference out=w191:refnum<vi>, error out=w190:errorcluster, "Value"=w123:dbl)  [unwired: 1 in]
          n87 = property class="DigNum (strict)"(reference=w187) -> (reference out=w188:refnum<vi>, error out=w189:errorcluster, "Value"=w186:dbl)  [unwired: 1 in]
          n88 = property class="DigNum (strict)"(reference=w184) -> (reference out=w182:refnum<vi>, error out=w183:errorcluster, "Value"=w181:dbl)  [unwired: 1 in]
          n89 = property class="DigNum (strict)"(reference=w178) -> (reference out=w180:refnum<vi>, error out=w179:errorcluster, "Value"=w171:dbl)  [unwired: 1 in]
          n90 = property class="DigNum (strict)"(reference=w177) -> (reference out=w175:refnum<vi>, error out=w176:errorcluster, "Value"=w170:dbl)  [unwired: 1 in]
          n91 = property class="DigNum (strict)"(reference=w173) -> (reference out=w169:refnum<vi>, error out=w174:errorcluster, "Value"=w168:dbl)  [unwired: 1 in]
          n92 = property class="DigNum (strict)"(reference=w166) -> (reference out=w167:refnum<vi>, error out=w165:errorcluster, "Value"=w164:dbl)  [unwired: 1 in]
          n93 = property class="DigNum (strict)"(reference=w162) -> (reference out=w161:refnum<vi>, error out=w163:errorcluster, "Value"=w148:dbl)  [unwired: 1 in]
          n94 = property class="DigNum (strict)"(reference=w159) -> (reference out=w160:refnum<vi>, error out=w158:errorcluster, "Value"=w147:dbl)  [unwired: 1 in]
          n95 = property class="DigNum (strict)"(reference=w153) -> (reference out=w146:refnum<vi>, error out=w154:errorcluster, "Value"=w145:dbl)  [unwired: 1 in]
          n96 = Close Reference(reference=w121, error in (no error)=w125) -> ()  [unwired: 1 out]
          n97 = property class="DigNum (strict)"(reference=w152) -> (reference out=w150:refnum<vi>, error out=w151:errorcluster, "Value"=w140:dbl)  [unwired: 1 in]
          n98 = property class="DigNum (strict)"(reference=w156) -> (reference out=w155:refnum<vi>, error out=w157:errorcluster, "Value"=w139:dbl)  [unwired: 1 in]
          n99 = call "ELAPSED TIMER VI FOR REPORT LOOP.vi"("TARGET"=w127, "RESET"=FALSE ("PAUSE"), "PAUSE"=w86) -> ("ELAPSED TIMER"=w194:dbl)  [unwired: 6 in, 2 out]
          n100 = Build Array(w194) -> (w120:dbl[])
          n101 = Divide(x=w124, y=w123) -> (x/y=w122:dbl)
          n102 = Close Reference(reference=w191, error in (no error)=w190) -> ()  [unwired: 1 out]
          n103 = Close Reference(reference=w188, error in (no error)=w189) -> ()  [unwired: 1 out]
          n104 = Close Reference(reference=w182, error in (no error)=w183) -> ()  [unwired: 1 out]
          n105 = Close Reference(reference=w180, error in (no error)=w179) -> ()  [unwired: 1 out]
          n106 = Close Reference(reference=w175, error in (no error)=w176) -> ()  [unwired: 1 out]
          n107 = Close Reference(reference=w169, error in (no error)=w174) -> ()  [unwired: 1 out]
          n108 = Close Reference(reference=w167, error in (no error)=w165) -> ()  [unwired: 1 out]
          n109 = Close Reference(reference=w161, error in (no error)=w163) -> ()  [unwired: 1 out]
          n110 = Close Reference(reference=w160, error in (no error)=w158) -> ()  [unwired: 1 out]
          n111 = Close Reference(reference=w146, error in (no error)=w154) -> ()  [unwired: 1 out]
          n112 = Close Reference(reference=w150, error in (no error)=w151) -> ()  [unwired: 1 out]
          n113 = Close Reference(reference=w155, error in (no error)=w157) -> ()  [unwired: 1 out]
          n114 = Divide(x=w186, y=w123) -> (x/y=w185:dbl)
          n115 = Not(x=w86) -> (.not. x?=w85:bool)
          n116 = Build Array(w123) -> (w119:dbl[])
          n117 = Build Array(w186) -> (w118:dbl[])
          n118 = Build Array(w185) -> (w117:dbl[])
          n119 = Build Array(w181) -> (w116:dbl[])
          n120 = Build Array(w172) -> (w115:dbl[])
          n121 = Build Array(w171) -> (w114:dbl[])
          n122 = Build Array(w170) -> (w113:dbl[])
          n123 = Build Array(w124) -> (w112:dbl[])
          n124 = Build Array(w122) -> (w111:dbl[])
          n125 = Build Array(w168) -> (w110:dbl[])
          n126 = Build Array(w164) -> (w109:dbl[])
          n127 = Build Array(w149) -> (w108:dbl[])
          n128 = Build Array(w148) -> (w107:dbl[])
          n129 = Build Array(w147) -> (w106:dbl[])
          n130 = Build Array(w145) -> (w105:dbl[])
          n131 = Build Array(w144) -> (w104:dbl[])
          n132 = Build Array(w143) -> (w103:dbl[])
          n133 = Build Array(w142) -> (w102:dbl[])
          n134 = Build Array(w141) -> (w101:dbl[])
          n135 = Build Array(w140) -> (w100:dbl[])
          n136 = Build Array(w139) -> (w99:dbl[])
          n137 = Build Array(w138) -> (w98:dbl[])
          n138 = Build Array(w137) -> (w97:dbl[])
          n139 = Build Array(w136) -> (w96:dbl[])
          n140 = Build Array(w135) -> (w95:dbl[])
          n141 = Build Array(w134) -> (w94:dbl[])
          n142 = Build Array(w133) -> (w93:dbl[])
          n143 = Build Array(w132) -> (w92:dbl[])
          n144 = Build Array(w131) -> (w91:dbl[])
          n145 = Insert Into Array(array=sgl[][] [], new element #1=w120, new element #2=w119, new element #3=w118, new element #4=w117, new element #5=w116, new element #6=w115, new element #7=w114, new element #8=w113, new element #9=w112, new element #10=w111, new element #11=w110, new element #12=w110, new element #13=w109, new element #14=w108, new element #15=w107, new element #16=w106, new element #17=w105, new element #18=w104, new element #19=w103, new element #20=w102, new element #21=w101, new element #22=w100, new element #23=w99, new element #24=w98, new element #25=w97, new element #26=w96, new element #27=w95, new element #28=w94, new element #29=w93, new element #30=w92, new element #31=w91) -> (w90:sgl[][])  [unwired: 2 in]
          n146 = case shown="True" w85 {
            tunnel: w90 -> [_ w207]
            frame False {
            }
            frame True {
              n147 = local read "tdms file out"() -> (w206:refnum<k34>)
              n148 = TDMS Write(0:w206, 5:"Measurement" ("group name in (Untitled)"), 7:string[] ["Time(Sec)", "Normal Load (N)", "Friction Force(N)", "Coefficient of Friction", " Depth (Microns)", "Speed (RPM0", "Frequency (Hz)", "Angle (Degree)", "Cyclic Friction Force (N)", "Cyclic Co-Efficient Friction Force", "Stage Temperature (Degree celcius)", "Sample Temperature (Degree celcius)", "Stroke Length (mm)", "Scratch Speed (mm/sec)", "Amb Humidity (%Rh)", "Amb Temperature (Deg C)", "Acoustic (mV)", "Mx(Nm)", "My(Nm);Mz(Nm)", "Humidity(%Rh)", "Sliding Distance (mm)", "Wear Track Diameter(mm)", "Fx(N)", "Fy(N)", "MTM Ball Speed(RPM)", "MTM Disc Speed (RPM)", "Entrainment Speed", "Slide Role", "Slip(%)"] ("array"), 9:w207) -> (4:w205:refnum<k34>)  [unwired: 2 in, 3 out]
              n149 = local write "tdms file out"(w205) -> ()
            }
          }
          "TDMS CLOSE" <- TRUE ("TDMS CLOSE")
        }
      }
    }
    frame Error {
    }
  }
